vi "check for new info.vi"(8 "error in (no error)":errorcluster, 9 "EOS":dbl, 10 "Spill ID":dbl, 11 "Beam in":refnum<class "Beam.lvclass">) -> (0 "error out":errorcluster, 3 "Beam out":refnum<class "Beam.lvclass">)   [LabVIEW 2019, in "Beam.lvclass"]
uses:
  Beam.lvclass
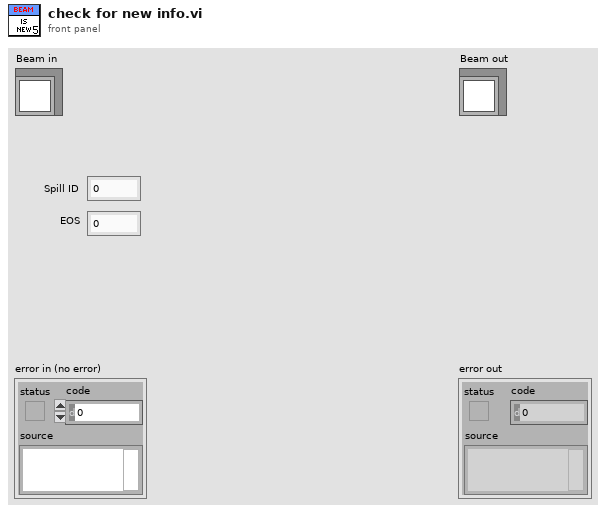
[diagram p1: front panel]
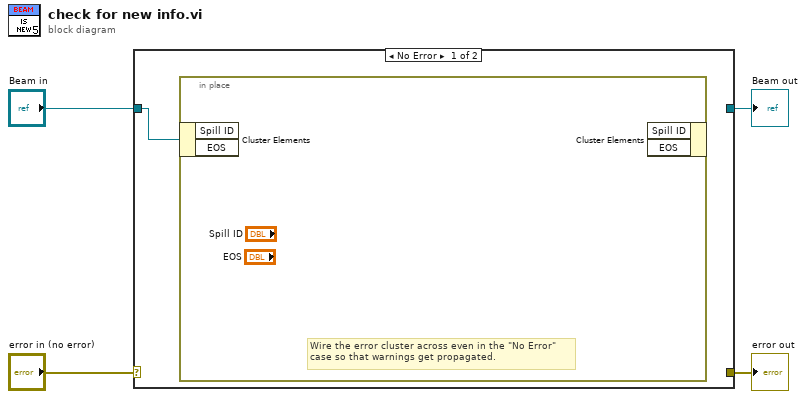
[diagram p0: block diagram]
diagram:
  n1 = case shown="No Error" "error in (no error)" {
    selector: "error in (no error)" -> [_ w7]
    tunnel: [_ w7] -> w3
    tunnel: [_ w6] -> w1
    tunnel: "Beam in" -> [w5 w6]
    frame No Error {
      n2 = in-place {
        # "Wire the error cluster across even in the \"No Error\"\ncase so that warnings get propagated."
        n3 = in-place-cluster #1(w5) -> ()  [unwired: 2 out]
        n4 = in-place-cluster #1() -> ()  [unwired: 2 in, 1 out]
      }
    }
    frame Error {
    }
  }
  "error out" <- w3
  "Beam out" <- w1
